vi "Formatta dati targa.vi"(8 "ItemNames DC":string[][](array[string]), 9 "RowHdrs[] DC":string[](array[string]), 10 "ItemNames DT":string[][](array[string]), 11 "RowHdrs[] DT":string[](array[string])) -> (3 "DATI TARGA":string[][](array[string]))   [LabVIEW 2019]
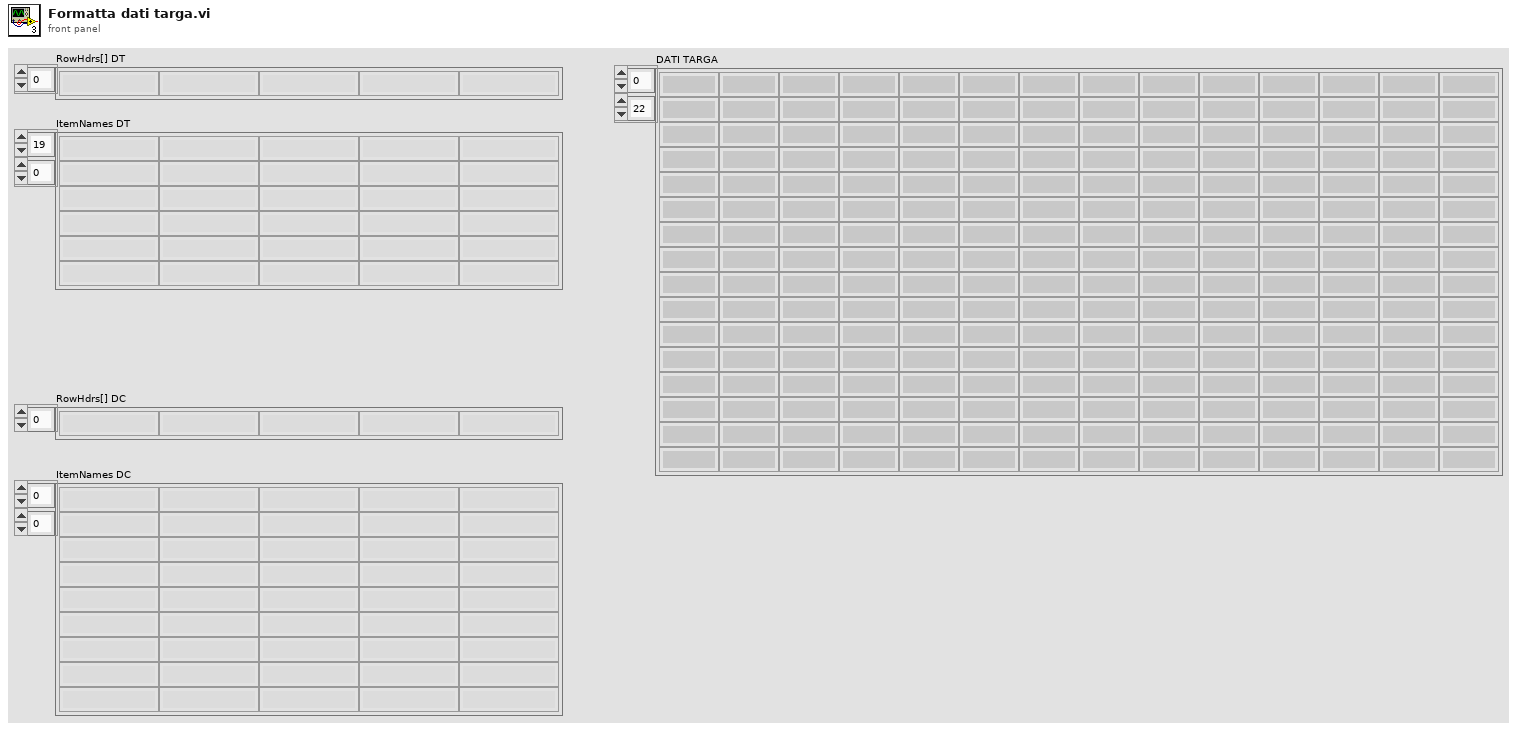
[diagram p1: front panel]
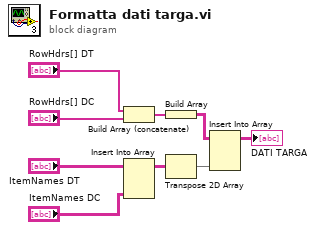
[diagram p0: block diagram]
diagram:
  n1 = Build Array (concatenate)("RowHdrs[] DT", "RowHdrs[] DC") -> (w4:string[])
  n2 = Insert Into Array(array="ItemNames DT", new element="ItemNames DC") -> (w8:string[][])  [unwired: 2 in]
  n3 = Build Array(w4) -> (w1:string[][])
  n4 = Transpose 2D Array(2D array=w8) -> (transposed array=w9:string[][])
  n5 = Insert Into Array(array=w1, new element=w9) -> (→"DATI TARGA":string[][])  [unwired: 2 in]
